vi "Show or Hide Spec Page Decorations.vi"(9 "Icon Visible":bool, 10 "Prefix Visible":bool, 11 "Spec Page refnum":refnum<vi>) -> ()   [LabVIEW 2016]
uses:
  <vilib>/UserTags/UserTags.lvlib
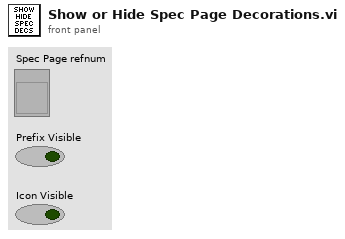
[diagram p1: front panel]
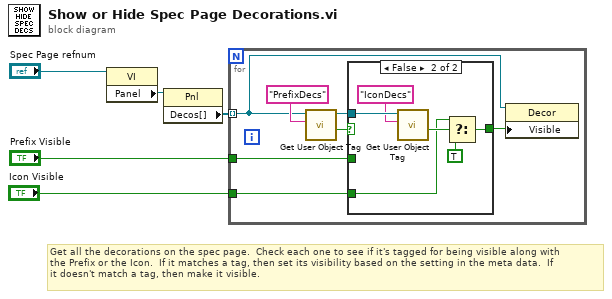
[diagram p0: block diagram]
diagram:
  # "Get all the decorations on the spec page.  Check each one to see if it's tagged for being visible along with\nthe Prefix or the Icon.  If it matches a tag, then set its visibility based on the setting in the meta data.  If\nit doesn't match a tag, then make it visible."
  n1 = property class="VI"(reference="Spec Page refnum") -> ("Panel"=w3:refnum<vi>)  [unwired: 1 in, 2 out]
  n2 = property class="Pnl"(reference=w3) -> ("Decos[]"=w5:refnum<vi>[])  [unwired: 1 in, 2 out]
  n3 = for {
    tunnel: w5 -> [w7] mode=indexing
    tunnel: "Prefix Visible" -> [w9]
    tunnel: "Icon Visible" -> [w8]
    n4 = call <vilib>:"Get User Object Tag.vi"("Tag Name"="PrefixDecs", "Generic Refnum"=w7) -> ("Was Tag Found?"=w11:bool, "dup Generic Refnum"=w10:refnum<vi>)  [unwired: 6 in, 2 out]
    n5 = case shown="False" w11 {
      tunnel: w10 -> [_ w19]
      tunnel: w9 -> [w13 _]
      tunnel: w8 -> [_ w16]
      tunnel: [w13 w14] -> w6
      frame True {
      }
      frame False {
        n6 = call <vilib>:"Get User Object Tag.vi"("Tag Name"="IconDecs", "Generic Refnum"=w19) -> ("Was Tag Found?"=w17:bool)  [unwired: 6 in, 3 out]
        n7 = Select(t=w16, s=w17, f=TRUE) -> (s? t:f=w14:bool)
      }
    }
    n8 = property class="Decor"(reference=w7, "Visible"=w6) -> ()  [unwired: 1 in, 2 out]
  }
